vi "Current Track Info.vi"(0 "reference in":refnum<class "MediaPlayer.lvclass">, 11 "Error In":errorcluster) -> (4 "reference out":refnum<class "MediaPlayer.lvclass">, 15 "Error Out":errorcluster)   [LabVIEW 2024, in "MediaPlayer.lvclass"]
doc: "Get Current track info.\n- Name (str)\n- Duration (DBL)"
uses:
  MediaPlayer.lvclass
  <vilib>/sound2/lvsound2.llb/Sound File Info (path).vi
  MediaPlayer.lvclass/MediaPlayer.ctl
panel:
  # "Connector Pane"
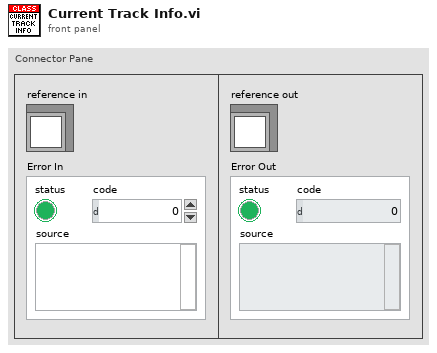
[diagram p1: front panel]
types:
  T1 = typedef "MediaPlayer.lvclass/ObjectAttributes.ctl" = cluster{"MediaPlayerData":T2, "Current Info":T4}
  T2 = typedef "MediaPlayer.lvclass/MediaPlayer Data.ctl" = cluster{"Music List":path[], "Current Music Index":i64, "Song Handler":T3, "Device ID":u32}
  T3 = typedef "Sound Output Task ID.ctl" = u32
  T4 = typedef "MediaPlayer.lvclass/Current Info.ctl" = cluster{"Duration":dbl, "Name":string, "Is playing?":bool, "Current Music Index":i64}
  T5 = typedef "Sound Data Format.ctl" = cluster{"sample rate (S/s)":dbl, "number of channels":i32, "bits per sample":i32}
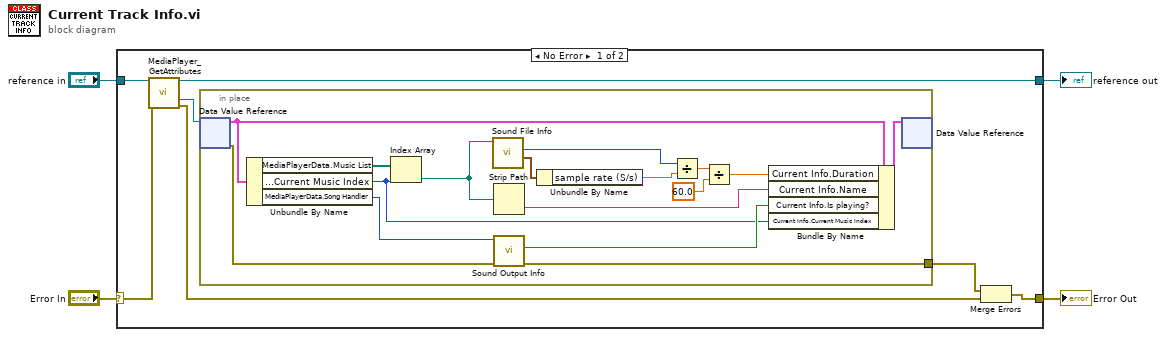
[diagram p0: block diagram]
diagram:
  n1 = case shown="No Error" "Error In" {
    selector: "Error In" -> [w11 w29]
    tunnel: [w6 w29] -> w3
    tunnel: [w9 w28] -> w1
    tunnel: "reference in" -> [w10 w28]
    frame No Error {
      n2 = call "MediaPlayer_GetAttributes.vi"("reference in"=w10, "Error In"=w11) -> ("reference out"=w9:refnum<class "MediaPlayer.lvclass">, "DataRef"=w8:refnum<data-value>, "Error Out"=w7:errorcluster)  [unwired: 10 in, 1 out]
      n3 = in-place {
        in-place-border: [w13] -> w5
        n4 = in-place-dvr #1(w8) -> (w19:T1, w14:errorcluster)
        n5 = Unbundle By Name(w19) -> ("MediaPlayerData.Music List"=w27:path[], "MediaPlayerData.Current Music Index"=w12:i64, "MediaPlayerData.Song Handler"=w26:T3)
        n6 = Index Array(array=w27, index=w12) -> (element=w25:path)
        n7 = call-poly <vilib>:"Sound File Info.vi"("path"=w25) -> ("sound format"=w24:T5, "total number of samples/ch"=w22:u32)  [unwired: 7 in, 2 out]
        n8 = Strip Path(path=w25) -> (name=w16:string)  [unwired: 1 out]
        n9 = call <vilib>:"Sound Output Info.vi"("error in (no error)"=w14, "task ID"=w26) -> ("error out"=w13:errorcluster, "is playing?"=w15:bool)  [unwired: 6 in, 2 out]
        n10 = Unbundle By Name(w24) -> ("sample rate (S/s)"=w23:dbl)
        n11 = Divide(x=w22, y=w23) -> (x/y=w21:dbl)
        n12 = Divide(x=w21, y=60.0) -> (x/y=w17:dbl)
        n13 = Bundle By Name(cluster=w19, "Current Info.Duration"=w17, "Current Info.Name"=w16, "Current Info.Is playing?"=w15, "Current Info.Current Music Index"=w12) -> (w18:T1)
        n14 = in-place-dvr #1(w18) -> ()  [unwired: 2 out]
      }
      n15 = Merge Errors(w5, w7) -> (w6:errorcluster)
    }
    frame Error {
    }
  }
  "Error Out" <- w3
  "reference out" <- w1
